vi "rs3 get frame number2.vi"(8 "error in (no error)":errorcluster, 11 "frame in":u64) -> (0 "error out":errorcluster, 1 "error":u64, 2 "Frame number":u64, 3 "frame out":u64)   [LabVIEW 2018, in "libRealSense3.lvlib"]
doc: "Provides timestamp"
uses:
  libRealSense3.lvlib
  realsense2.dll
panel:
  # "RS3 Get Frame Number"
  # "(C) Intel Corp.,  AGJ"
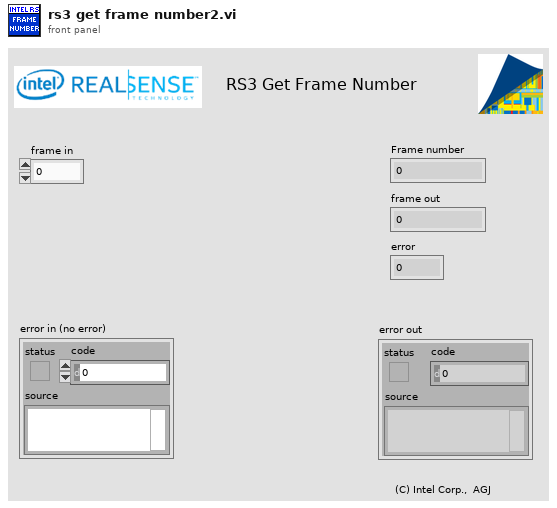
[diagram p1: front panel]
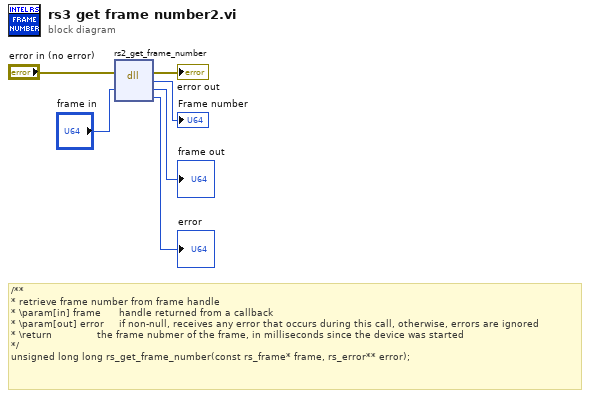
[diagram p0: block diagram]
diagram:
  # "/**\n* retrieve frame number from frame handle\n* \\param[in] frame      handle returned from a callback\n* \\param[out] error     if non-null, receives any error that occurs during this call, otherwise, errors are ignored\n* \\return               the frame nubmer of the frame, in milliseconds since the device was started\n*/\nunsigned long long rs_get_frame_number(const rs_frame* frame, rs_error** error);"
  n1 = dll-call lib="C:/Users/aaron.jencks/Documents/GitHub/emerson_seed_object_detection/LabVIEW/Projects/Paul's Video Viewer/Classes/Realsense Cam/realsense_wrapper_api/realsense2.dll" fn="rs2_get_frame_number"(error in="error in (no error)", "frame"="frame in") -> (error out=→"error out":errorcluster, "frame number"=→"Frame number":u64, "frame"=→"frame out":u64, "error"=→"error":u64)  [unwired: 3 in, 1 out]
